vi "MyFunPath1.vi"() -> (4 "path":cluster{"X":dbl, "Y":dbl}[](array[cluster])=[{"X"=68.0, "Y"=162.0}, {"X"=173.13402061855672, "Y"=174.98257839721256}, {"X"=234.37113402061857, "Y"=250.62020905923347}, {"X"=237.71134020618558, "Y"=265.2961672473868}, {"X"=237.15463917525773, "Y"=271.50522648083626}])   [LabVIEW 2018]
uses:
  AutonBuilder/Typedef/Data Point.ctl
panel:
  in  "Data Points":T1[](array[typedef])=[{"X"=68.0, "Y"=162.0, "Theta"=0.0, "Speed %"=0.0, "Disabled?"=FALSE}, {"X"=173.13402061855672, "Y"=174.98257839721256, "Theta"=0.0, "Speed %"=0.0, "Disabled?"=FALSE}, {"X"=234.37113402061857, "Y"=250.62020905923347, "Theta"=0.0, "Speed %"=0.0, "Disabled?"=FALSE}, {"X"=237.71134020618558, "Y"=265.2961672473868, "Theta"=0.0, "Speed %"=0.0, "Disabled?"=FALSE}, {"X"=237.15463917525773, "Y"=271.50522648083626, "Theta"=0.0, "Speed %"=0.0, "Disabled?"=FALSE}]
  out "Graph":cluster{dbl[], dbl[]}[](graph)=[{[0.0, 33.5, 33.5, 0.0, 0.0], [176.25, 176.25, 147.75, 147.75, 176.25]}, {[68.0, 173.13402061855672, 234.37113402061857, 237.71134020618558, 237.15463917525773], [162.0, 174.98257839721256, 250.62020905923347, 265.2961672473868, 271.50522648083626]}, {array[228 elements], array[228 elements]}, {array[228 elements], array[228 elements]}, {array[228 elements], array[228 elements]}, {[], []}, {[], []}, {[], []}, {[], []}, {[], []}]
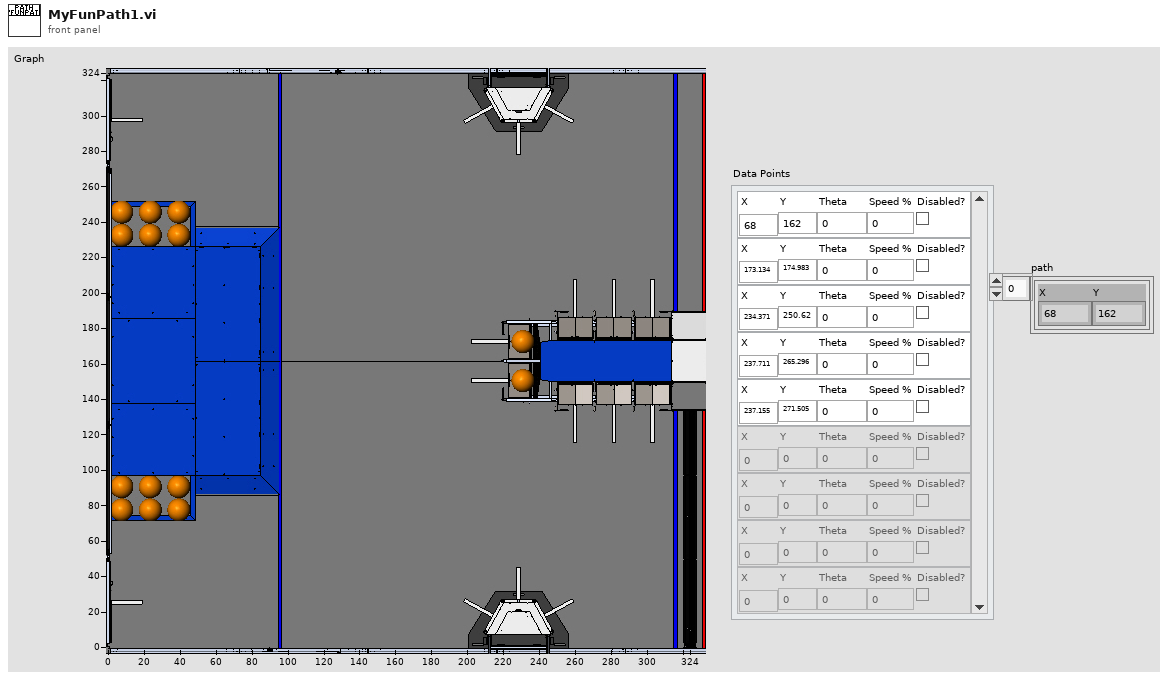
[diagram p1: front panel]
types:
  T1 = typedef "Data Point.ctl" = cluster{"X":dbl, "Y":dbl, "Theta":dbl, "Speed %":dbl, "Disabled?":bool}
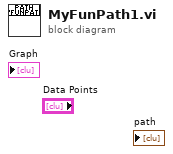
[diagram p0: block diagram]
diagram:
